vi "Index Traj2Joint Output.vi"(8 "Deform Array":dbl[](array[numeric])=[1.0, 1.0, 1.0, 0.0, 0.0, 0.0, 0.0, 0.0, 0.0], 9 "Pivot Pt":dbl[](array[numeric])=[0.0, 5.0, 0.0], 10 "Index":i32, 11 "Trajectory Cluster":T1) -> (1 "Indexed Cart Posit":dbl[](array[numeric]), 3 "Indexed Joit Posit":dbl[](array[numeric]))   [LabVIEW 2016]
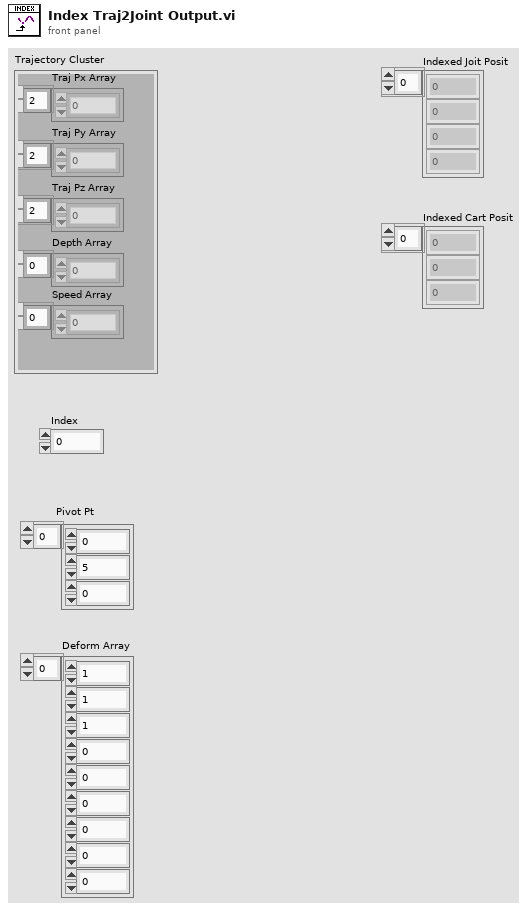
[diagram p1: front panel]
types:
  T1 = cluster{"Traj Px Array":dbl[], "Traj Py Array":dbl[], "Traj Pz Array":dbl[], "Speed Array":dbl[], "Depth Array":dbl[]}
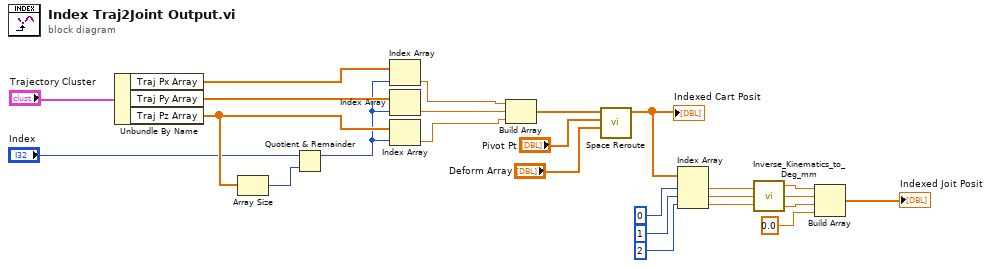
[diagram p0: block diagram]
diagram:
  n1 = Unbundle By Name("Trajectory Cluster") -> ("Traj Px Array"=w21:dbl[], "Traj Py Array"=w25:dbl[], "Traj Pz Array"=w19:dbl[])
  n2 = Array Size(array=w19) -> (size(s)=w18:i32)
  n3 = Quotient & Remainder(x="Index", y=w18) -> (x-y*floor(x/y)=w17:i32)  [unwired: 1 out]
  n4 = Index Array(array=w21, index=w17) -> (element=w24:dbl)
  n5 = Index Array(array=w25, index=w17) -> (element=w23:dbl)
  n6 = Index Array(array=w19, index=w17) -> (element=w22:dbl)
  n7 = Build Array(w24, w23, w22) -> (w15:dbl[])
  n8 = call "Space Reroute.vi"("Deform Array"="Deform Array", "Pivot Pt"="Pivot Pt", "Nominal Traj Pt"=w15) -> ("Reroute Traj Pt"=w2:dbl[])  [unwired: 8 in]
  "Indexed Cart Posit" <- w2
  n9 = Index Array(array=w2, index #1=0 ("index"), index #2=1 ("index"), index #3=2 ("index")) -> (element #1=w7:dbl, element #2=w5:dbl, element #3=w6:dbl)
  n10 = call "Inverse_Kinematics_to_Deg_mm.vi"("pz"=w6, "py"=w5, "px"=w7) -> ("L3 [mm]"=w10:dbl, "L2 [deg]"=w9:dbl, "L1 [deg]"=w8:dbl)
  n11 = Build Array(w8, w9, w10, 0.0 ("element")) -> (→"Indexed Joit Posit":dbl[])
